vi "Charge_meas.vi"() -> ()   [LabVIEW 2018]
uses:
  <instrlib>/AFG-2225/AFG-2225.lvlib
panel:
  in  "stop":bool
  in  "Delay Time (s)":dbl=1.0
  in  "Field Time (s)":dbl=1.0 caption="Delay Time (s)"
  in  "DC Offset (0.00 V)":dbl format="%.2g"
  in  "Frequency (1000.000 Hz)":dbl=1000.0 format="%_7g"
  in  "Amplitude (3.000 Vpp)":dbl=3.0 format="%.3g"
  in  "Waveform Function (0: Sine)":u16(ring) items=["Sine", "Square", "Pulse", "Ramp", "Noise"]
  in  "Impedance (0: 50 OHM)":u16(ring) items=["50 OHM", "High Z"]
  in  "Channel (0: CH1)":u16(ring) items=["CH1", "CH2"]
  # "Wait for a loop to end then stop"
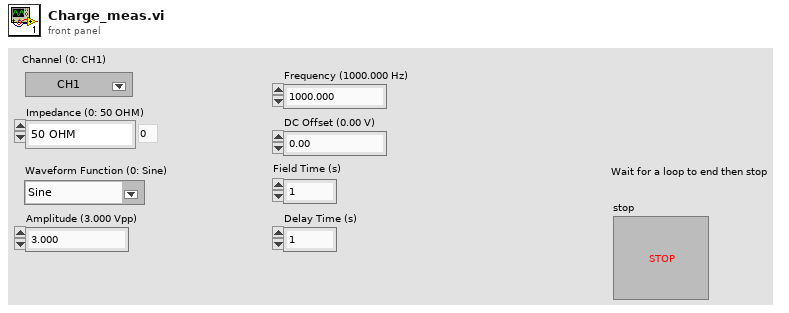
[diagram p1: front panel]
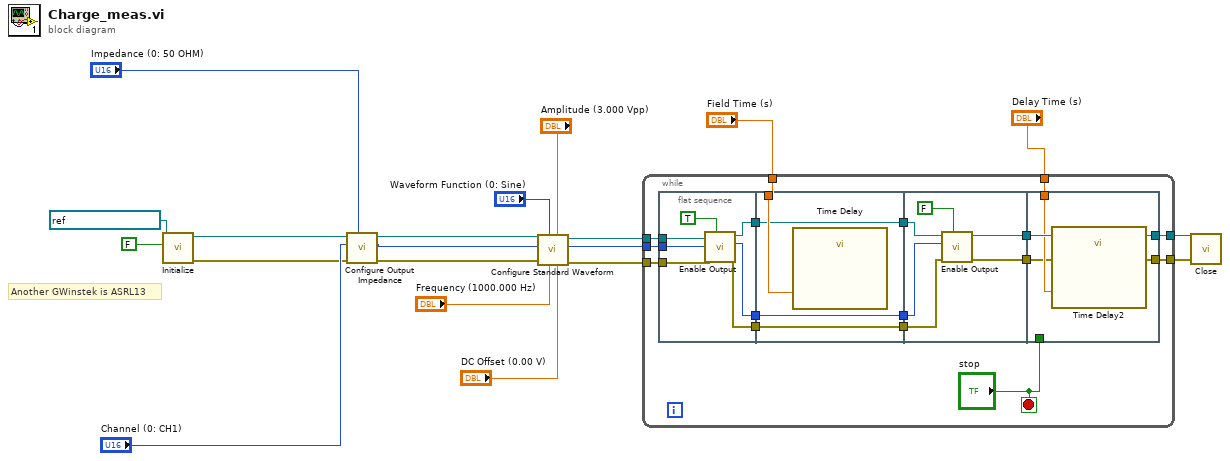
[diagram p0: block diagram]
diagram:
  # "Another GWinstek is ASRL13"
  n1 = call <instrlib>:"Initialize.vi"("ID Query (True)"=FALSE, "VISA resource name"=refnum<visa-resource-name> "AFG2225SYNTH") -> ("error out"=w16:errorcluster, "VISA resource name out"=w17:refnum<visa-resource-name>)  [unwired: 8 in]
  n2 = call <instrlib>:"Configure Output Impedance.vi"("VISA resource name"=w17, "Channel (0: CH1)"="Channel (0: CH1)", "error in (no error)"=w16, "Impedance (0: 50 OHM)"="Impedance (0: 50 OHM)") -> ("VISA resource name out"=w14:refnum<visa-resource-name>, "Channel out"=w12:u16, "error out"=w13:errorcluster)  [unwired: 4 in]
  n3 = call <instrlib>:"Configure Standard Waveform.vi"("DC Offset (0.00 V)"="DC Offset (0.00 V)", "Amplitude (3.000 Vpp)"="Amplitude (3.000 Vpp)", "Frequency (1000.000 Hz)"="Frequency (1000.000 Hz)", "Waveform Function (0: Sine)"="Waveform Function (0: Sine)", "error in (no error)"=w13, "Channel (0: CH1)"=w12, "VISA resource name"=w14) -> ("error out"=w5:errorcluster, "Channel out"=w6:u16, "VISA resource name out"=w7:refnum<visa-resource-name>)  [unwired: 2 in]
  n4 = while {
    tunnel: w7 -> [w36]
    tunnel: w6 -> [w35]
    tunnel: w5 -> [w34]
    tunnel: "Field Time (s)" -> [w33]
    tunnel: [w26] -> w3
    tunnel: [w25] -> w2
    tunnel: "Delay Time (s)" -> [w22]
    stop <- "stop" stop-if-true
    n5 = flat-sequence {
      tunnel: w36 -> [w43]
      tunnel: w35 -> [w42]
      tunnel: w34 -> [w41]
      tunnel: [w39] -> w31
      tunnel: [w38] -> w29
      tunnel: [w37] -> w27
      tunnel: w33 -> [w47]
      tunnel: [w46] -> w32
      tunnel: w31 -> [w46]
      tunnel: [w45] -> w30
      tunnel: w29 -> [w45]
      tunnel: [w44] -> w28
      tunnel: w27 -> [w44]
      tunnel: w32 -> [w53]
      tunnel: w30 -> [w52]
      tunnel: w28 -> [w51]
      tunnel: [w50] -> w24
      tunnel: [w49] -> w23
      tunnel: [w56] -> w25
      tunnel: [w54] -> w26
      tunnel: w24 -> [w54]
      tunnel: w23 -> [w56]
      tunnel: w22 -> [w55]
      tunnel: "stop" -> [_]
      frame #0 {
        n6 = call <instrlib>:"Enable Output.vi"("Enable Output (T: Enable)"=TRUE, "error in (no error)"=w41, "Channel (0: CH1)"=w42, "VISA resource name"=w43) -> ("error out"=w37:errorcluster, "Channel out"=w38:u16, "VISA resource name out"=w39:refnum<visa-resource-name>)  [unwired: 5 in]
      }
      frame #1 {
        n7 = call "Time Delay"("Delay Time (s)"=w47) -> ()  [unwired: 10 in, 1 out]
      }
      frame #2 {
        n8 = call <instrlib>:"Enable Output.vi"("Enable Output (T: Enable)"=FALSE, "error in (no error)"=w51, "Channel (0: CH1)"=w52, "VISA resource name"=w53) -> ("error out"=w50:errorcluster, "VISA resource name out"=w49:refnum<visa-resource-name>)  [unwired: 5 in, 1 out]
      }
      frame #3 {
        n9 = call "Time Delay2"("Delay Time (s)"=w55) -> ()  [unwired: 10 in, 1 out]
      }
    }
  }
  n10 = call <instrlib>:"Close.vi"("error in (no error)"=w3, "VISA resource name"=w2) -> ()  [unwired: 9 in, 1 out]
